vi "DAQmx Read (Digital 1D U32 NChan 1Samp).vi"(0 "task/channels in":refnum<k21>, 9 "timeout":dbl=10.0 format="%0.2f", 11 "error in":errorcluster) -> (4 "task out":refnum<k21>, 6 "data":u32[](array[numeric]), 15 "error out":errorcluster)   [LabVIEW 2024]
doc: "Reads a single 32-bit unsigned integer sample from each channel in a task that contains one or more digital input channels. Use an instance that reads 32-bit unsigned integers for devices with up to 32 lines per port."
uses:
  nilvaiu.dll
panel:
  # "channel"
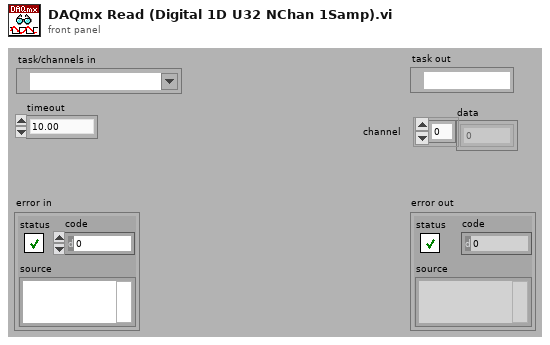
[diagram p1: front panel]
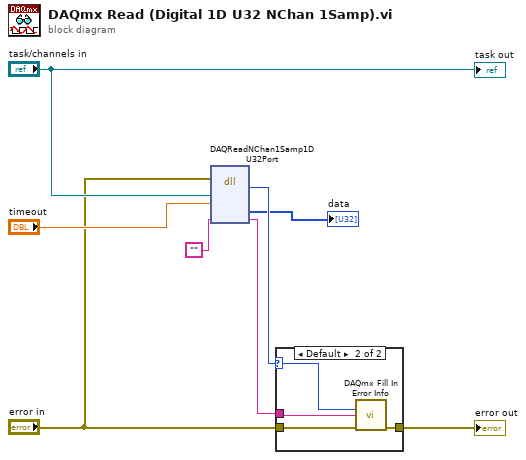
[diagram p0: block diagram]
diagram:
  n1 = dll-call lib="nilvaiu.*" fn="DAQReadNChan1Samp1DU32Port"(error in="error in", "taskID"="task/channels in", "timeout"="timeout", "extendedErrorInfo"="") -> ("return type"=w6:i32, "data"=→"data":u32[], "extendedErrorInfo"=w4:string)  [unwired: 4 in, 3 out]
  n2 = case shown="Default" w6 {
    selector: w6 -> [_ w11]
    tunnel: "error in" -> [w9 w13]
    tunnel: [w9 w12] -> w8
    tunnel: w4 -> [_ w10]
    frame 0 {
    }
    frame Default {
      n3 = call "DAQmx Fill In Error Info.vi"("status code"=w11, "extended error info"=w10, "error in"=w13) -> ("error out"=w12:errorcluster)  [unwired: 1 in, 11 out]
    }
  }
  "error out" <- w8
  "task out" <- "task/channels in"
